vi "Z-scan_v3.vi"() -> ()   [LabVIEW 2010]
uses:
  <vilib>/express/express arith-compare/Formula/XNode/ExpressFormulaBlockNode.xnode
  <vilib>/DAQmx/read.llb/DAQmx Read (Analog 1D Wfm NChan NSamp).vi
  <vilib>/daqmx/miscellaneous.llb/DAQmx Fill In Error Info.vi
  <vilib>/express/express shared/transition.llb/Dynamic To Waveform Array.vi
  <vilib>/express/express shared/transition.llb/Waveform Array To Dynamic.vi
  <vilib>/express/express arith-compare/Formula/Block/exnFormulaBlock how many pts in the wave.vi
  <vilib>/express/express shared/ex_Modify Signal Name.vi
panel:
  out "Signal 3":dbl[][](graph)
  out "Ioa":cluster{dbl[], dbl[]}(graph)
  out "Ica":cluster{dbl[], dbl[]}(graph)
  out "Ioca":cluster{dbl[], dbl[]}(graph)
  in  "stop 11":bool
  in  "lower threshold":dbl
  in  "upper threshold":dbl
  in  "z max (mm)":dbl=500.0
  in  "z step (mm)":dbl=5.0
  in  "Acquisition time (s)":i32=1000
  in  "z min (mm)":dbl=-0.5
  in  "CURSOR":u16(ring)=1 items=["Ref", "CA", "OA"]
  in  "stop 2":bool
  out "Signal 2":waveform(dbl)[](graph)
  in  "error in 2":errorcluster
  in  "STOP":bool
  in  "Z-SCAN":bool
  in  "PHOTODIODE SIGNALS":bool
  in  "INITIALIZE":bool
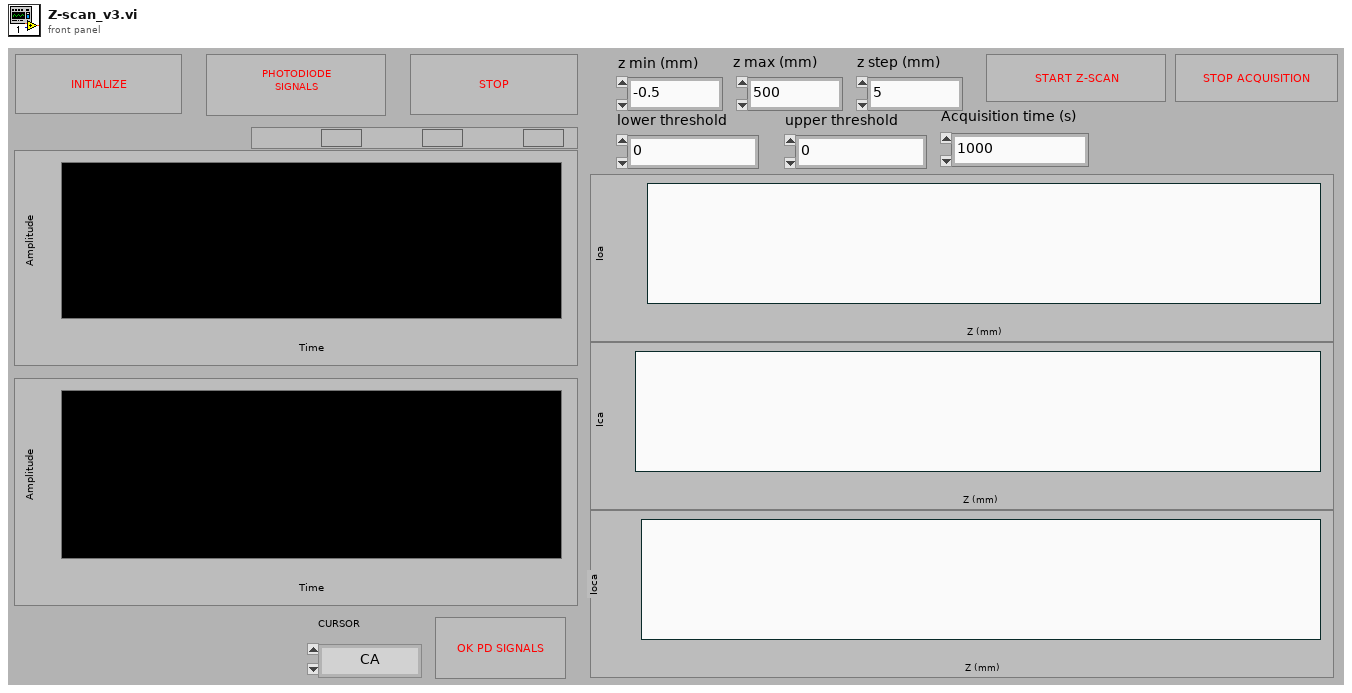
[diagram p1: front panel]
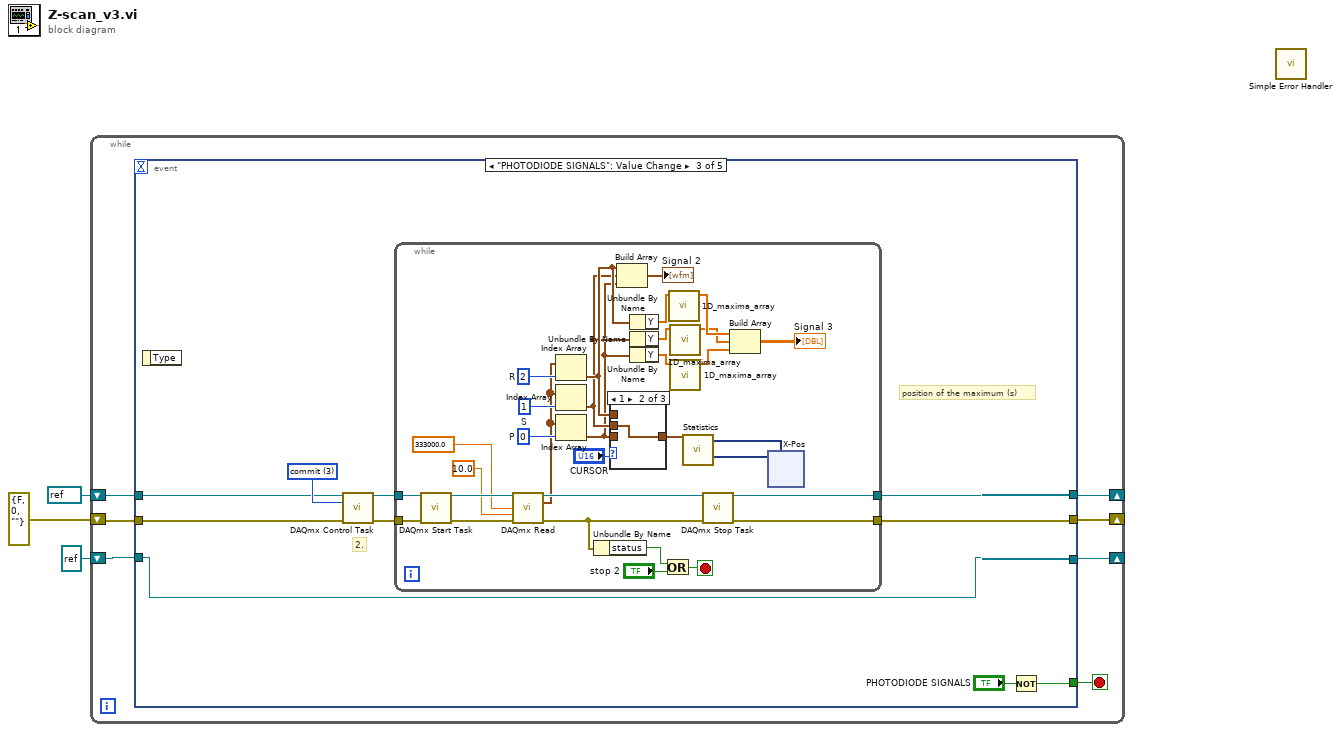
[diagram p0: block diagram]
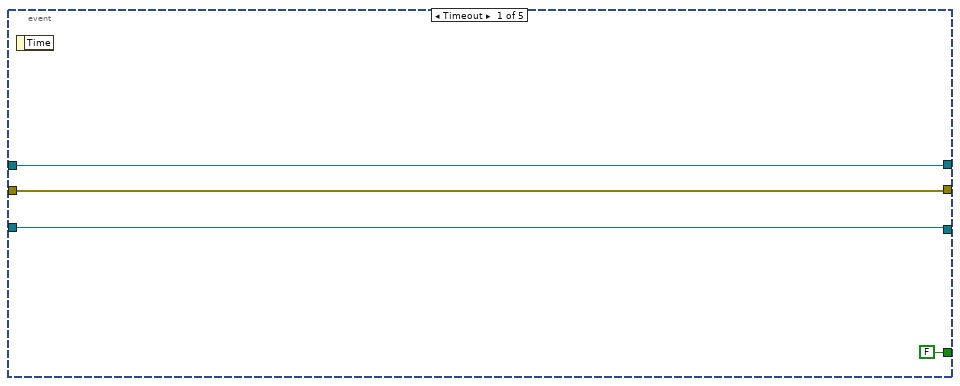
[diagram p2: hidden frame]
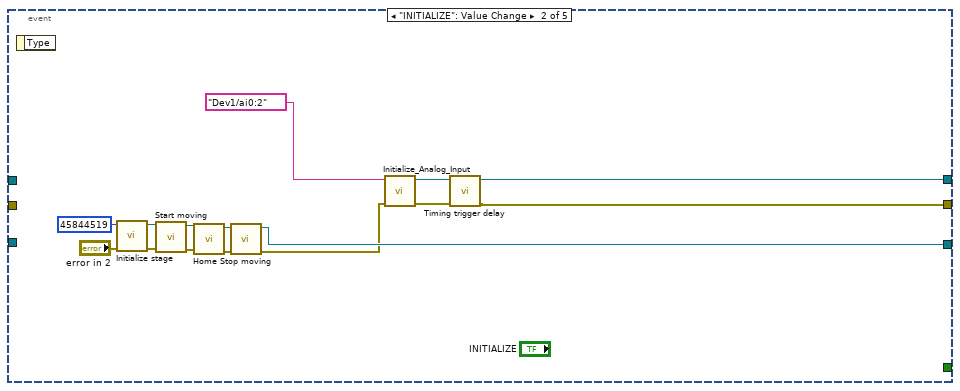
[diagram p3: hidden frame]
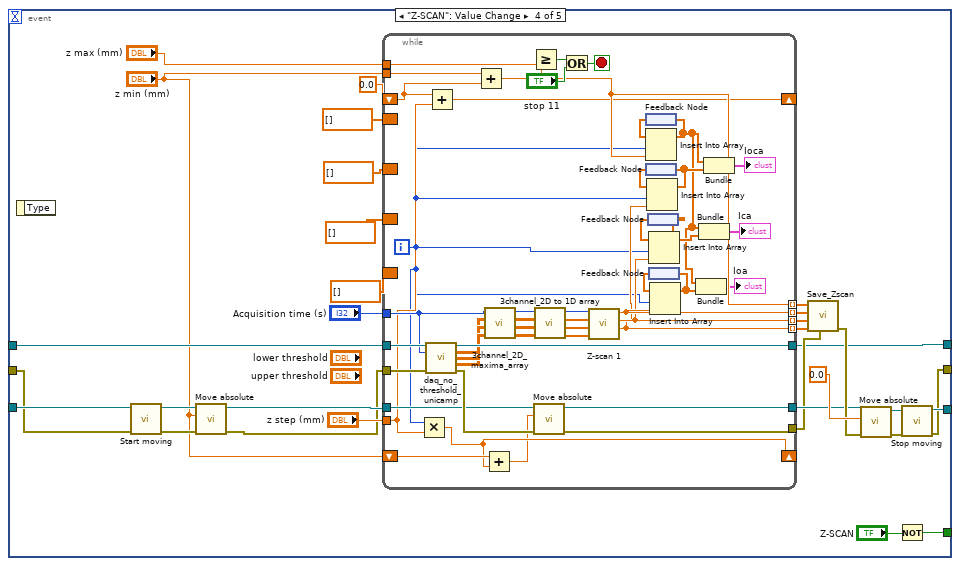
[diagram p6: hidden frame]
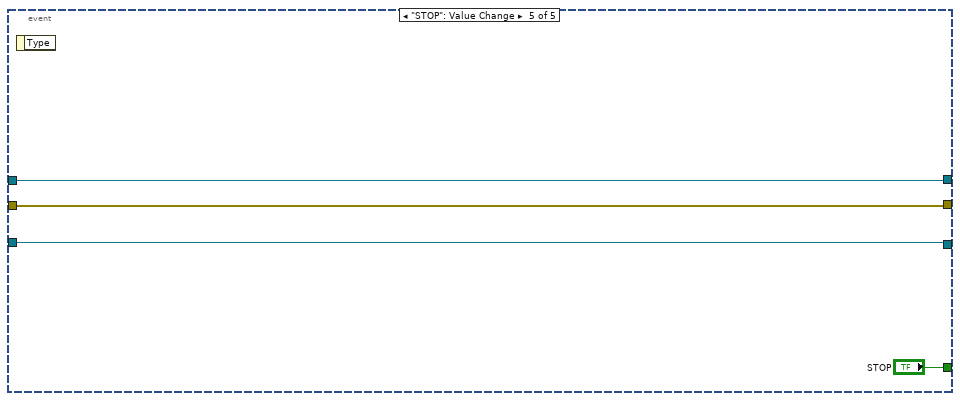
[diagram p7: hidden frame]
diagram:
  n1 = while {
    shift-right: [w9] -> _
    shift-left: refnum<k21> refnum ("task out") -> [w6]
    shift-right: [w8] -> _
    shift-left: errorcluster {"status"=FALSE, "code"=0, "source"=""} ("error out") -> [w4]
    shift-right: [w7] -> _
    shift-left: refnum<k7> refnum ("Motor out") -> [w5]
    stop <- w10 stop-if-true
    n2 = event shown="[2] \"PHOTODIODE SIGNALS\": Value Change" {
      selector: _ -> [_ _ _ _ _]
      dyn-events: _ -> [_ _ _ _ _]
      timeout: _ -> [_ _ _ _ _]
      tunnel: [FALSE ("STOP") _ w31 w215 "STOP"] -> w10
      tunnel: [w12 w16 w34 w222 w291] -> w9
      tunnel: [w13 w15 w33 w214 w292] -> w8
      tunnel: [w14 w21 w32 w224 w293] -> w7
      tunnel: w6 -> [w12 _ w36 w225 w291]
      tunnel: w5 -> [w14 _ w32 w221 w293]
      tunnel: w4 -> [w13 _ w35 w219 w292]
      event Timeout {
        n3 = event-data() -> ()  [unwired: 1 in, 1 out]
      }
      event "INITIALIZE": Value Change {
        n4 = event-data() -> ()  [unwired: 1 in, 1 out]
        n5 = call <userlib>:"Initialize stage.vi"("error in (no error)"="error in 2", "HWSerialNum"=45844519) -> ("error out"=w25:errorcluster, "reference out"=w27:refnum<k7>)  [unwired: 8 in]
        n6 = call <userlib>:"Start moving.vi"("error in (no error)"=w25, "Motor in"=w27) -> ("error out"=w24:errorcluster, "Motor out"=w26:refnum<k7>)  [unwired: 8 in]
        n7 = call <userlib>:"Home.vi"("error in"=w24, "in"=w26) -> ("error out"=w22:errorcluster, "out"=w23:refnum<k7>)  [unwired: 8 in]
        n8 = call <userlib>:"Stop moving.vi"("error in (no error)"=w22, "Motor in"=w23) -> ("error out"=w19:errorcluster, "Motor out"=w21:refnum<k7>)  [unwired: 8 in]
        n9 = call <userlib>:"Initialize_Analog_Input.vi"("error in"=w19, "Channels"=tag "Dev1/ai0:2" ("Signal")) -> ("error out"=w17:errorcluster, "task out"=w18:refnum<k21>)  [unwired: 8 in]
        n10 = call <userlib>:"Timing trigger delay.vi"("error in"=w17, "task/channels in"=w18) -> ("error out"=w15:errorcluster, "task out"=w16:refnum<k21>)  [unwired: 8 in]
      }
      event "PHOTODIODE SIGNALS": Value Change {
        w39 = 3 items=["verify"=2, "reserve"=4, "commit"=3, "unreserve"=5, "abort"=6] ("action")
        # "position of the maximum (s)"
        # "2."
        n11 = event-data() -> ()  [unwired: 1 in, 1 out]
        n12 = call <vilib>:"DAQmx Control Task.vi"("task/channels in"=w36, "action"=w39, "error in"=w35) -> ("task out"=w38:refnum<k21>, "error out"=w37:errorcluster)  [unwired: 11 in]
        n13 = while {
          tunnel: w38 -> [w71]
          tunnel: w37 -> [w70]
          tunnel: [w55] -> w33
          tunnel: [w50] -> w34
          stop <- w51 stop-if-true
          w63 = 0  # P
          w64 = 1  # S
          w65 = 2  # R
          n14 = call <vilib>:"DAQmx Start Task.vi"("task/channels in"=w71, "error in"=w70) -> ("task out"=w69:refnum<k21>, "error out"=w68:errorcluster)  [unwired: 12 in]
          n15 = call-poly <vilib>:"DAQmx Read.vi"("task/channels in"=w69, "number of samples per channel"=333000.0 ("Samples/channel"), "timeout"=10.0, "error in"=w68) -> ("task out"=w67:refnum<k21>, "data"=w62:waveform(dbl)[], "error out"=w53:errorcluster)  [unwired: 9 in]
          n16 = Index Array(array=w62, index=w65) -> (element=w49:waveform(dbl))
          n17 = Index Array(array=w62, index=w64) -> (element=w48:waveform(dbl))
          n18 = Index Array(array=w62, index=w63) -> (element=w47:waveform(dbl))
          n19 = Unbundle By Name(w53) -> ("status"=w54:bool)
          n20 = case shown="1" "CURSOR" {
            tunnel: w47 -> [w211 _ _]
            tunnel: [w211 w212 w213] -> w58
            tunnel: w48 -> [_ w212 _]
            tunnel: w49 -> [_ _ w213]
            frame 0, Default {
            }
            frame 1 {
            }
            frame 2 {
            }
          }
          n21 = Build Array(w49, w48, w47) -> (→"Signal 2":waveform(dbl)[])
          n22 = Unbundle By Name(w49) -> ("Y"=w46:dbl[])
          n23 = Unbundle By Name(w48) -> ("Y"=w45:dbl[])
          n24 = Unbundle By Name(w47) -> ("Y"=w44:dbl[])
          n25 = Or(x=w54, y="stop 2") -> (x .or. y?=w51:bool)
          n26 = call <userlib>:"1D_maxima_array.vi"("Array in"=w46) -> ("Array out"=w43:dbl[])  [unwired: 7 in, 3 out]
          n27 = call <userlib>:"1D_maxima_array.vi"("Array in"=w45) -> ("Array out"=w42:dbl[])  [unwired: 7 in, 3 out]
          n28 = call <userlib>:"1D_maxima_array.vi"("Array in"=w44) -> ("Array out"=w41:dbl[])  [unwired: 7 in, 3 out]
          n29 = call "Statistics"("Signals"=w58) -> ("First Time"=w59:dynamicdata, "Time of Maximum"=w60:dynamicdata)  [unwired: 21 in, 4 out]
          n30 = call <vilib>:"DAQmx Stop Task.vi"("task/channels in"=w67, "error in"=w53) -> ("task out"=w50:refnum<k21>, "error out"=w55:errorcluster)  [unwired: 12 in]
          n31 = Build Array(w43, w42, w41) -> (→"Signal 3":dbl[][])
          n32 = xnode "X-Pos"("TimeMax"=w60, "1stTime"=w59) -> ()  [unwired: 1 in, 2 out]
        }
        n33 = Not(x="PHOTODIODE SIGNALS") -> (.not. x?=w31:bool)
      }
      event "Z-SCAN": Value Change {
        n34 = event-data() -> ()  [unwired: 1 in, 1 out]
        n35 = call <userlib>:"Start moving.vi"("error in (no error)"=w219, "Motor in"=w221) -> ("error out"=w244:errorcluster, "Motor out"=w243:refnum<k7>)  [unwired: 8 in]
        n36 = call <userlib>:"Move absolute.vi"("error in (no error)"=w244, "target position"="z min (mm)", "Motor in"=w243) -> ("error out"=w218:errorcluster, "Motor out"=w220:refnum<k7>)  [unwired: 7 in]
        n37 = while {
          tunnel: "z max (mm)" -> [w288]
          tunnel: [w274] -> w239
          tunnel: "z min (mm)" -> [w284]
          tunnel: "z step (mm)" -> [w248]
          shift-right: [w273] -> _
          shift-left: 0.0 -> [w283]
          border: dbl[] [] -> [_]
          border: dbl[] [] -> [_]
          border: dbl[] [] -> [_]
          border: dbl[] [] -> [_]
          tunnel: [w276] -> w235 mode=indexing
          tunnel: [w269] -> w236 mode=indexing
          tunnel: [w268] -> w237 mode=indexing
          tunnel: [w267] -> w238 mode=indexing
          tunnel: [w266] -> w240
          tunnel: w225 -> [w265]
          tunnel: w220 -> [w264]
          tunnel: w218 -> [w263]
          tunnel: "Acquisition time (s)" -> [w258]
          tunnel: [w262] -> w222
          shift-right: [w246] -> _
          shift-left: "z min (mm)" -> [w249]
          i -> [w247]
          stop <- w286 stop-if-true
          n38 = Multiply(x=w247, y=w248) -> (x*y=w246:dbl)
          n39 = call <userlib>:"daq_no_threshold_unicamp.vi"("channels in"=w265, "Acquisition time (s)"=w258, "error in"=w263) -> ("task out"=w262:refnum<k21>, "REF"=w261:dbl[][], "OA"=w260:dbl[][], "CA"=w259:dbl[][], "error out"=w275:errorcluster)  [unwired: 8 in]
          n40 = Add(x=w283, y=w248) -> (x+y=w273:dbl)
          n41 = Add(x=w284, y=w283) -> (x+y=w276:dbl)
          n42 = Add(x=w249, y=w246) -> (x+y=w245:dbl)
          n43 = call <userlib>:"3channel_2D_maxima_array.vi"("2D Reference array"=w261, "2D OA array"=w260, "2D CA array"=w259, "Acquisition time (s)"=w258) -> ("2D maxima reference array"=w254:dbl[][], "2D maxima OA array"=w255:dbl[][], "2D maxima CA array"=w256:dbl[][], "Acquisition time (s) 2"=w257:i32)  [unwired: 4 in]
          n44 = Greater Or Equal?(x=w276, y=w288) -> (x >= y?=w287:bool)
          n45 = call <userlib>:"Move absolute.vi"("error in (no error)"=w275, "target position"=w245, "Motor in"=w264) -> ("error out"=w274:errorcluster, "Motor out"=w266:refnum<k7>)  [unwired: 7 in]
          n46 = call <userlib>:"3channel_2D to 1D array.vi"("2D maxima reference array in"=w254, "2D maxima OA array in"=w255, "2D maxima CA array in"=w256, "Acquisition time (s)"=w257) -> ("1D reference array out"=w251:dbl[], "1D OA array out"=w252:dbl[], "1D CA array out"=w253:dbl[], "Acquisition time (s)"=w250:i32)  [unwired: 4 in]
          n47 = Or(x=w287, y="stop 11") -> (x .or. y?=w286:bool)
          n48 = call <userlib>:"Z-scan 1.vi"("Ref"=w251, "CA"=w252, "OA"=w253, "Acquisition time (s)"=w250) -> ("Ioca"=w267:dbl, "Ica"=w268:dbl, "Ioa"=w269:dbl)  [unwired: 3 in]
          n49 = feedback #1() -> (w279:dbl[])
          n50 = Insert Into Array(array=w279, index=w247, new element=w276) -> (w272:dbl[])
          n51 = feedback-in #1(w272) -> ()
          n52 = feedback #2() -> (w278:dbl[])
          n53 = Insert Into Array(array=w278, index=w247, new element=w267) -> (w280:dbl[])
          n54 = feedback-in #2(w280) -> ()
          n55 = feedback #3() -> (w282:dbl[])
          n56 = Insert Into Array(array=w282, index=w247, new element=w268) -> (w281:dbl[])
          n57 = feedback-in #3(w281) -> ()
          n58 = feedback #4() -> (w290:dbl[])
          n59 = Insert Into Array(array=w290, index=w247, new element=w269) -> (w289:dbl[])
          n60 = feedback-in #4(w289) -> ()
          n61 = Bundle(w272, w289) -> (→"Ioa":cluster{dbl[], dbl[]})  [unwired: 1 in]
          n62 = Bundle(w272, w281) -> (→"Ica":cluster{dbl[], dbl[]})  [unwired: 1 in]
          n63 = Bundle(w272, w280) -> (→"Ioca":cluster{dbl[], dbl[]})  [unwired: 1 in]
        }
        n64 = call "Save_Zscan.vi"("error in"=w239, "Ioca"=w238, "Ica"=w237, "Ioa"=w236, "z (mm)"=w235) -> ("error out"=w241:errorcluster)  [unwired: 6 in]
        n65 = call <userlib>:"Move absolute.vi"("error in (no error)"=w241, "target position"=sgl 0.0 ("Set absolute position"), "Motor in"=w240) -> ("error out"=w226:errorcluster, "Motor out"=w227:refnum<k7>)  [unwired: 7 in]
        n66 = Not(x="Z-SCAN") -> (.not. x?=w215:bool)
        n67 = call <userlib>:"Stop moving.vi"("error in (no error)"=w226, "Motor in"=w227) -> ("error out"=w214:errorcluster, "Motor out"=w224:refnum<k7>)  [unwired: 8 in]
      }
      event "STOP": Value Change {
        n68 = event-data() -> ()  [unwired: 1 in, 1 out]
      }
    }
  }
  n69 = call <vilib>:"Simple Error Handler.vi"() -> ()  [unwired: 2 in, 8 out]
